vi "Generic_3DPrinter_2.vi"() -> ()   [LabVIEW 2010]
panel:
  in  "VISA resource name":refnum<visa-resource-name>="COM1"
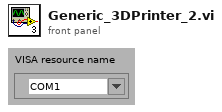
[diagram p1: front panel]
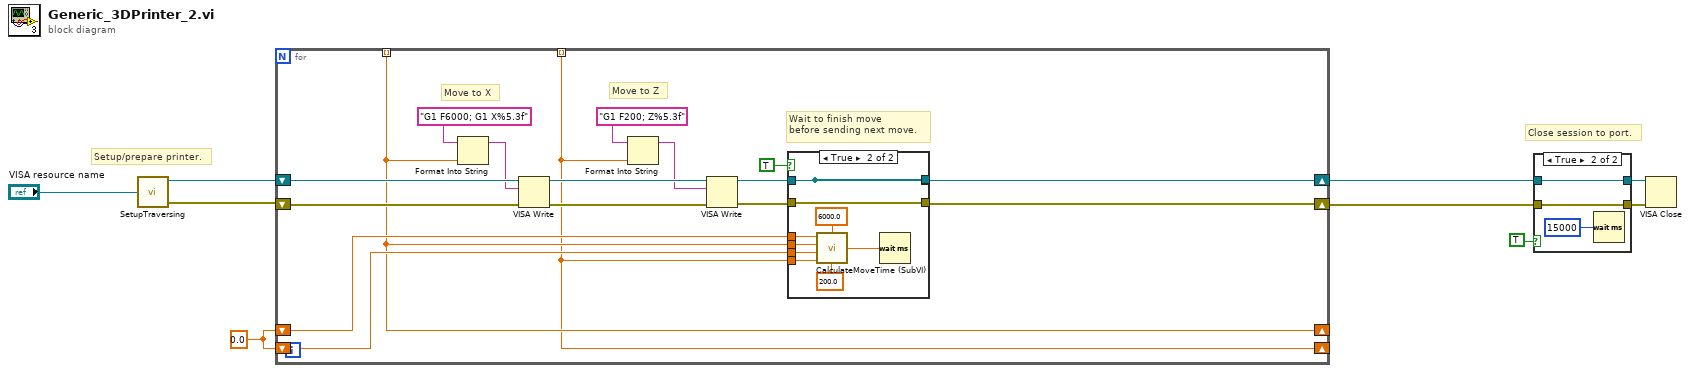
[diagram p0: block diagram]
diagram:
  w3 = 0.0
  # "Setup/prepare printer."
  # "Close session to port."
  n1 = call "SetupTraversing.vi"("VISA resource name"="VISA resource name") -> ("error out"=w5:errorcluster, "VISA resource name out"=w6:refnum<visa-resource-name>)
  n2 = for {
    tunnel: _ -> [w11] mode=indexing
    tunnel: _ -> [w10] mode=indexing
    shift-right: [w15] -> w2
    shift-left: w6 -> [w26]
    shift-right: [w14] -> w1
    shift-left: w5 -> [w25]
    shift-right: [w11] -> _
    shift-left: w3 -> [w13]
    shift-right: [w10] -> _
    shift-left: w3 -> [w12]
    # "Wait to finish move \nbefore sending next move."
    # "Move to Z"
    # "Move to X"
    n3 = Format Into String(initial string="G1 F6000; G1 X%5.3f" ("string to write 4"), w11) -> (resulting string=w18:string)  [unwired: 2 in, 1 out]
    n4 = VISA Write(VISA resource name=w26, write buffer=w18, error in (no error)=w25) -> (VISA resource name out=w24:refnum<visa-resource-name>, error out=w23:errorcluster)  [unwired: 1 out]
    n5 = Format Into String(initial string="G1 F200; Z%5.3f" ("string to write 4"), w10) -> (resulting string=w22:string)  [unwired: 2 in, 1 out]
    n6 = VISA Write(VISA resource name=w24, write buffer=w22, error in (no error)=w23) -> (VISA resource name out=w20:refnum<visa-resource-name>, error out=w19:errorcluster)  [unwired: 1 out]
    n7 = case shown="True" TRUE ("write") {
      tunnel: [w27 w37] -> w14
      tunnel: [w28 w36] -> _
      tunnel: w20 -> [w28 w36]
      tunnel: w19 -> [w27 w37]
      tunnel: [_ w36] -> w15
      tunnel: w13 -> [_ w32]
      tunnel: w12 -> [_ w31]
      tunnel: w11 -> [_ w30]
      tunnel: w10 -> [_ w29]
      frame False {
      }
      frame True {
        n8 = call "CalculateMoveTime (SubVI).vi"("ZSpeed(mm/min)"=200.0, "XSpeed (mm/min)"=6000.0, "New Z"=w29, "Previous Z"=w31, "New X"=w30, "Previous X"=w32) -> ("Adjusted Time(s)"=w35:dbl)
        n9 = Wait (ms)(milliseconds to wait=w35) -> ()  [unwired: 1 out]
      }
    }
  }
  n10 = case shown="True" TRUE ("write") {
    tunnel: [w38 w41] -> w8
    tunnel: [w39 w40] -> w7
    tunnel: w2 -> [w39 w40]
    tunnel: w1 -> [w38 w41]
    frame False {
    }
    frame True {
      n11 = Wait (ms)(milliseconds to wait=u32 15000) -> ()  [unwired: 1 out]
    }
  }
  n12 = VISA Close(VISA resource name=w7, error in (no error)=w8) -> ()  [unwired: 1 out]
